vi "RP Logic Specs.vi"(11 "Logic tag":u16) -> (0 "Number of output channels":i32, 1 "Number of  input channels":i32, 2 "Bytes per sample":i32, 3 "Samples per trigger increment":i32, 4 "Check RAM":bool, 5 "DC Gain":dbl=1.0, 6 "DC address increment":i32)   [LabVIEW 2024]
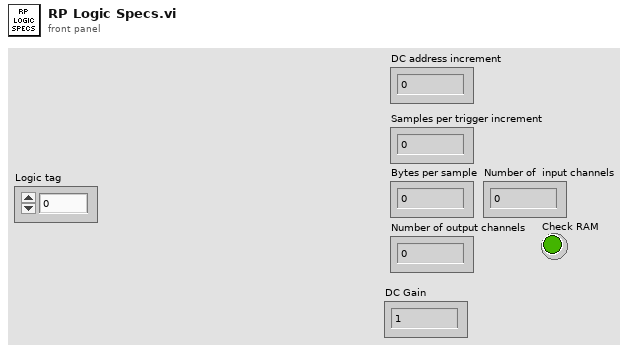
[diagram p1: front panel]
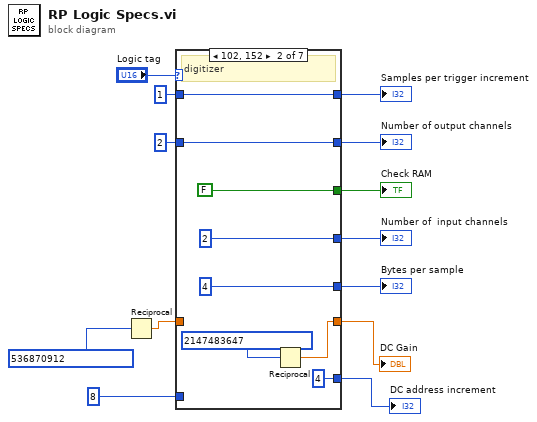
[diagram p0: block diagram]
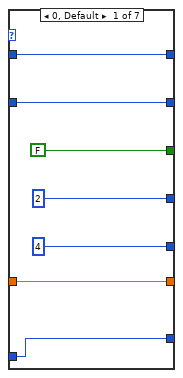
[diagram p2: hidden frame]
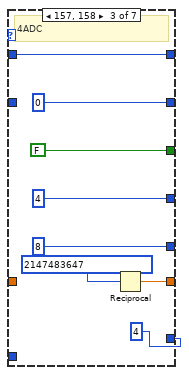
[diagram p3: hidden frame]
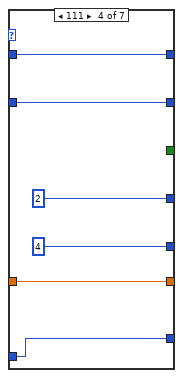
[diagram p4: hidden frame]
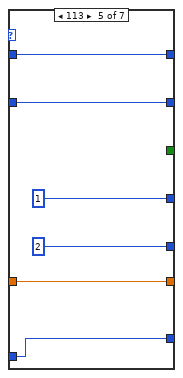
[diagram p5: hidden frame]
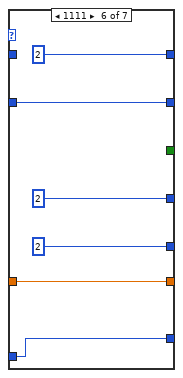
[diagram p6: hidden frame]
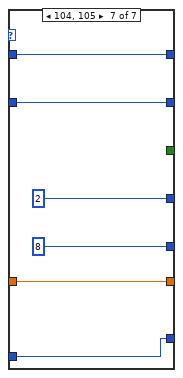
[diagram p7: hidden frame]
diagram:
  n1 = Reciprocal(x=536870912) -> (1/x=w3:dbl)
  n2 = case shown="102, 152" "Logic tag" {
    tunnel: [4 ("Trigger granularity") 4 ("Trigger granularity") 8 ("Trigger granularity") 4 ("Trigger granularity") 2 ("Trigger granularity") 2 ("Trigger granularity") 8 ("Trigger granularity")] -> w10
    tunnel: 1 ("Samples per trigger increment") -> [w19 w27 w35 w41 w47 _ w59]
    tunnel: [w19 w27 w35 w41 w47 2 ("Samples per trigger increment") w59] -> w11
    tunnel: [2 ("Trigger granularity") 2 ("Trigger granularity") 4 ("Trigger granularity") 2 ("Trigger granularity") 1 ("Trigger granularity") 2 ("Trigger granularity") 2 ("Trigger granularity")] -> w9
    tunnel: 2 ("Samples per trigger increment") -> [w17 w25 _ w39 w45 w51 w57]
    tunnel: [w17 w25 0 ("Samples per trigger increment") w39 w45 w51 w57] -> w8
    tunnel: [FALSE FALSE FALSE _ _ _ _] -> w7
    tunnel: [w15 w21 w30 w38 w44 w50 w56] -> w5
    tunnel: w3 -> [w15 _ _ w38 w44 w50 w56]
    tunnel: [w14 4 ("Samples per trigger increment") 4 ("Samples per trigger increment") w37 w43 w49 w55] -> w1
    tunnel: 8 ("Samples per trigger increment") -> [w14 _ _ w37 w43 w49 w55]
    frame 0, Default {
    }
    frame 102, 152 {
      # "digitizer"
      n3 = Reciprocal(x=2147483647) -> (1/x=w21:dbl)
    }
    frame 157, 158 {
      # "4ADC"
      n4 = Reciprocal(x=2147483647) -> (1/x=w30:dbl)
    }
    frame 111 {
    }
    frame 113 {
    }
    frame 1111 {
    }
    frame 104, 105 {
    }
  }
  "Samples per trigger increment" <- w11
  "Bytes per sample" <- w10
  "Number of  input channels" <- w9
  "Number of output channels" <- w8
  "Check RAM" <- w7
  "DC Gain" <- w5
  "DC address increment" <- w1
